vi "HP3457_MeasureDUTVoltage.vi"(7 "error in":errorcluster) -> (0 "error out":errorcluster, 2 "DUTVoltage":dbl)   [LabVIEW 2020]
panel:
  out "return count 2nd read":u32
  out "return count 1st read":u32
  out "First read data":string
  # "ORIGINAL : 40"
  # "ORIGINAL : 40"
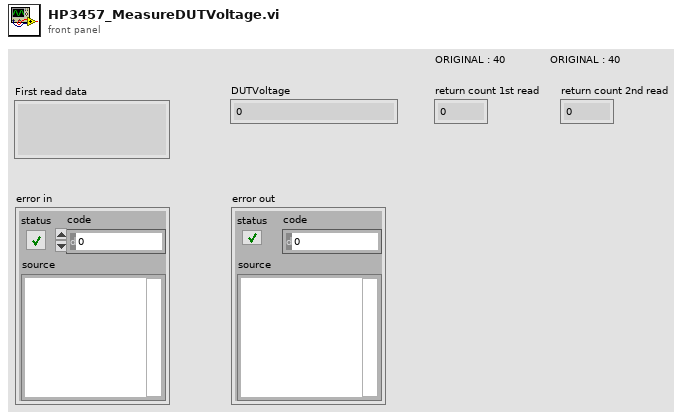
[diagram p1: front panel]
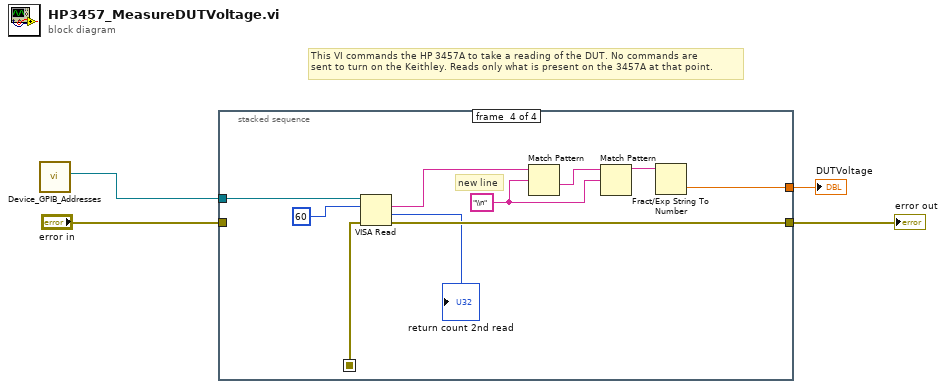
[diagram p0: block diagram]
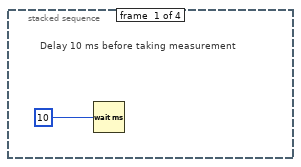
[diagram p2: hidden frame]
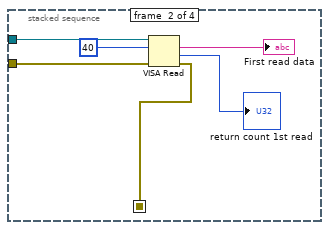
[diagram p3: hidden frame]
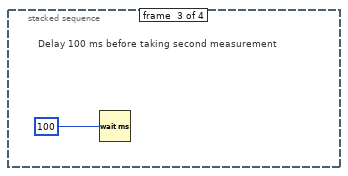
[diagram p4: hidden frame]
diagram:
  # "This VI commands the HP 3457A to take a reading of the DUT. No commands are\nsent to turn on the Keithley. Reads only what is present on the 3457A at that point."
  n1 = call "Device_GPIB_Addresses.vi"() -> ("HP 3457A Address"=w1:refnum<visa-resource-name>)  [unwired: 9 in, 2 out]
  n2 = stacked-sequence {
    seq-local: [_ w8 _ _] -> [_ _ _ w16]
    tunnel: w1 -> [_ w7 _ w18]
    tunnel: "error in" -> [_ w9 _ _]
    tunnel: [_ _ _ w14] -> w3
    tunnel: [_ _ _ w20] -> w2
    frame #0 {
      # "Delay 10 ms before taking measurement"
      n3 = Wait (ms)(milliseconds to wait=u32 10) -> ()  [unwired: 1 out]
    }
    frame #1 {
      n4 = VISA Read(VISA resource name=w7, byte count=40, error in (no error)=w9) -> (read buffer=→"First read data":string, return count=→"return count 1st read":u32, error out=w8:errorcluster)  [unwired: 1 out]
    }
    frame #2 {
      # "Delay 100 ms before taking second measurement"
      n5 = Wait (ms)(milliseconds to wait=u32 100) -> ()  [unwired: 1 out]
    }
    frame #3 {
      w21 = "\\n" ("regular expression")
      # "new line"
      n6 = VISA Read(VISA resource name=w18, byte count=60, error in (no error)=w16) -> (read buffer=w15:string, return count=→"return count 2nd read":u32, error out=w14:errorcluster)  [unwired: 1 out]
      n7 = Match Pattern(string=w15, regular expression=w21) -> (after substring=w22:string)  [unwired: 1 in, 3 out]
      n8 = Match Pattern(string=w22, regular expression=w21) -> (before substring=w19:string)  [unwired: 1 in, 3 out]
      n9 = Fract/Exp String To Number(string=w19) -> (number=w20:dbl)  [unwired: 3 in, 1 out]
    }
  }
  "error out" <- w3
  "DUTVoltage" <- w2
